vi "output.vi"(8 "error in":errorcluster, 10 "data table in":T1, 11 "Profibus Module runtime in":refnum<class "Profibus Module runtime.lvclass">) -> (0 "error out":errorcluster, 2 "data table out":T1, 3 "Profibus Module runtime out":refnum<class "Profibus Module runtime.lvclass">)   [LabVIEW 2013, in "Profibus Module runtime.lvclass"]
doc: "Provides an interface for writing data to a module at runtime. While this interface performs no operations, a child should provide an override which may write to any open sessions, references, or interfaces."
uses:
  Profibus Module runtime.lvclass
  <vilib>/addons/Comsoft.lib/cRIO PBMS/CS_cRIO-PB_DP-Master_FPGA-Reference.ctl
  <vilib>/NI/Tag Bus/table/data table.ctl
  <vilib>/NI/Tag Bus/table/data table.lvlib
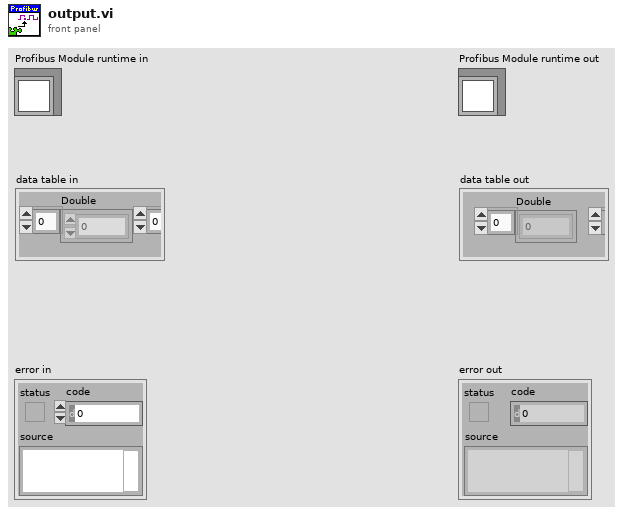
[diagram p1: front panel]
types:
  T1 = typedef "tag bus.lvlib/data table.lvlib/data table.ctl" = cluster{"Double":dbl[], "Single":sgl[], "I64":i64[], "I32":i32[], "I16":i16[], "I8":i8[], "U64":u64[], "U32":u32[], "U16":u16[], "U8":u8[], "Boolean":bool[], "String":string[], "Array of Double":cluster{"DBL Array":dbl[]}[], "Array of Single":cluster{"SGL Array":sgl[]}[], "Array of I64":cluster{"I64 Array":i64[]}[], "Array of I32":cluster{"I32 Array":i32[]}[], "Array of I16":cluster{"I16 Array":i16[]}[], "Array of I8":cluster{"I8 Array":i8[]}[], "Array of U64":cluster{"U64 Array":u64[]}[], "Array of U32":cluster{"U32 Array":u32[]}[], "Array of U16":cluster{"U16 Array":u16[]}[], "Array of U8":cluster{"U8 Array":u8[]}[], "Array of Boolean":cluster{"Boolean Array":bool[]}[], "Array of String":cluster{"String Array":string[]}[]}
  T2 = typedef "CS_cRIO-PB_DP-Master_FPGA-Reference.ctl" = refnum<k20>
  T3 = typedef "Profibus Module runtime.lvclass/profibus slave configuration.ctl" = cluster{"slave index":i8, "data items":T4[], "data buffer":u8[]}
  T4 = typedef "Profibus Module runtime.lvclass/profibus mapping configuration.ctl" = cluster{"data type":T5, " byte":i32, " bit":i32, "tag index":i32}
  T5 = typedef "tag bus.lvlib/tag descriptor.lvclass/Data Type.ctl" = enum16{"Double", "Single", "I64", "I32", "I16", "I8", "U64", "U32", "U16", "U8", "Boolean", "String", "Array of Double", "Array of Single", "Array of I64", "Array of I32", "Array of I16", "Array of I8", "Array of U64", "Array of U32", "Array of U16", "Array of U8", "Array of Boolean", "Array of String"}
  T6 = enum16{"Start/Stop DP-Master", "Get Input Data", "Set Output Data", "Get Output Data", "Get Diagnostic Data", "Read/Write Data", "Read Diagnostic Data", "Get DPV1 Data", "Set DPV1 Data", "Read/Write DPV1 Data"}
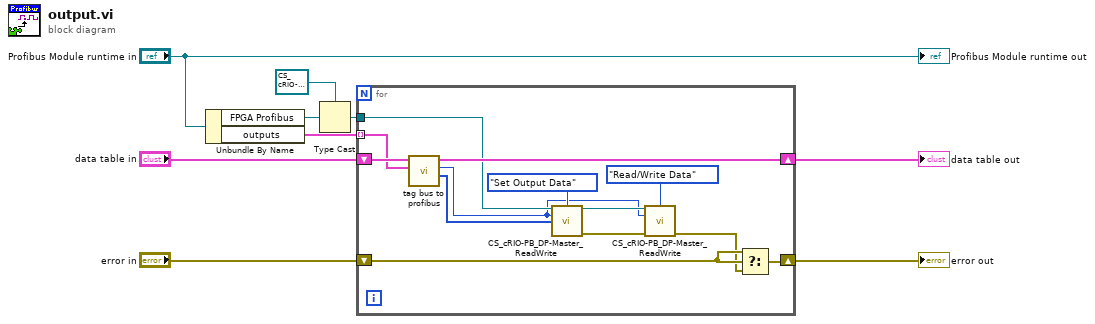
[diagram p0: block diagram]
diagram:
  n1 = Unbundle By Name("Profibus Module runtime in") -> ("FPGA Profibus"=w3:refnum<k20>, "outputs"=w7:T3[])
  n2 = Type Cast(type=T2 refnum ("FPGA VI Reference out"), x=w3) -> (*(type *) &x=w2:T2)
  n3 = for {
    shift-right: [w21] -> w8
    shift-left: "data table in" -> [w22]
    tunnel: w7 -> [w19] mode=indexing
    shift-right: [w16] -> w4
    shift-left: "error in" -> [w15]
    tunnel: w2 -> [w17]
    n4 = call "tag bus to profibus.vi"("slave configuration"=w19, "data table in in"=w22) -> ("Data"=w20:u8[], "slave index"=w10:i8, "data table out"=w21:T1)  [unwired: 7 in]
    n5 = call <vilib>:"CS_cRIO-PB_DP-Master_ReadWrite.vi"("FPGA VI Reference"=w17, "Mode"=T6."Set Output Data", "Slave"=w10, "Data"=w20) -> ("FPGA VI Reference out"=w11:T2, "Error out"=w13:errorcluster)  [unwired: 8 in, 2 out]
    n6 = call <vilib>:"CS_cRIO-PB_DP-Master_ReadWrite.vi"("FPGA VI Reference"=w11, "Mode"=T6."Read/Write Data", "Slave"=w10, "Error"=w13) -> ("Error out"=w12:errorcluster)  [unwired: 8 in, 3 out]
    n7 = Select(t=w15, s=w15, f=w12) -> (s? t:f=w16:errorcluster)
  }
  "error out" <- w4
  "data table out" <- w8
  "Profibus Module runtime out" <- "Profibus Module runtime in"
